vi "CleanUp.vi"(8 "error in (no error)":errorcluster, 11 "Prueba21 in":refnum<class "Prueba21.lvclass">) -> (0 "error out":errorcluster, 3 "Prueba21 out":refnum<class "Prueba21.lvclass">)   [LabVIEW 2019, in "Prueba21.lvclass"]
uses:
  Prueba21.lvclass
  C:/Users/ivan_/Documents/procal/Pruebas/Prueba/Prueba.lvclass
  Prueba/Prueba.lvclass/Prueba.ctl
  Prueba21.lvclass/Prueba21.ctl
  Base de Datos/SQLiteConnector/SQLiteConnection.lvclass
  Base de Datos/Base de Datos.lvclass
  Prueba/Prueba.lvclass
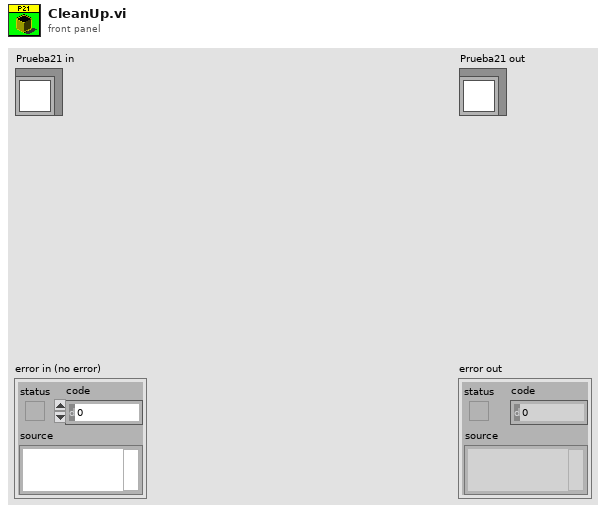
[diagram p1: front panel]
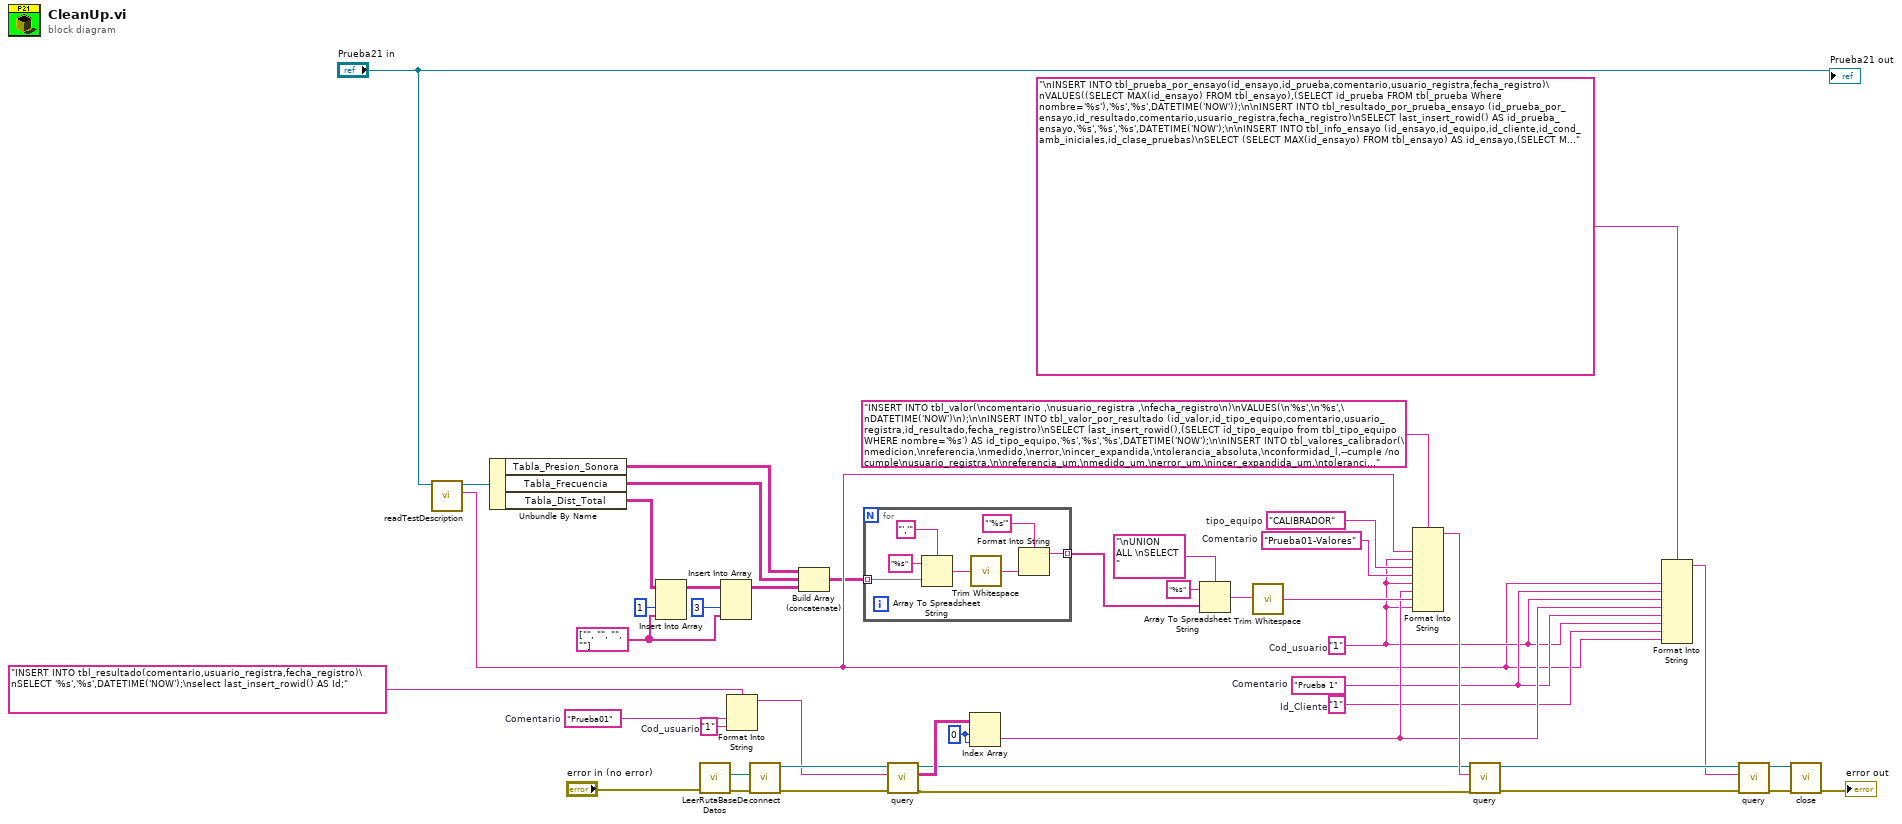
[diagram p0: block diagram]
diagram:
  w3 = string[] ["", "", "", ""]
  w18 = "1"  # Id_Cliente
  w19 = "Prueba 1"  # Comentario
  w28 = "CALIBRADOR"  # tipo_equipo
  w27 = "Prueba01-Valores"  # Comentario
  w33 = 0 ("index (row)")
  w35 = "1"  # Cod_usuario
  w36 = "Prueba01"  # Comentario
  w17 = "1"  # Cod_usuario
  n1 = call "readTestDescription.vi"("Prueba in"="Prueba21 in") -> ("Test Description"=w14:string, "Prueba out"=w15:refnum<class "Prueba21.lvclass">)  [unwired: 8 in, 1 out]
  n2 = Unbundle By Name(w15) -> ("Tabla_Presion_Sonora"=w8:string[][], "Tabla_Frecuencia"=w9:string[][], "Tabla_Dist_Total"=w2:string[][])
  n3 = Insert Into Array(array=w2, index (col)=1 ("disabled index (col)"), new element=w3) -> (w4:string[][])  [unwired: 1 in]
  n4 = call "LeerRutaBaseDeDatos.vi"("error in (no error)"="error in (no error)") -> ("error out"=w40:errorcluster, "Database Path"=w39:path)  [unwired: 9 in]
  n5 = Insert Into Array(array=w4, index (col)=3 ("disabled index (col)"), new element=w3) -> (w1:string[][])  [unwired: 1 in]
  n6 = Format Into String(format string="INSERT INTO tbl_resultado(comentario,usuario_registra,fecha_registro)\nSELECT '%s','%s',DATETIME('NOW');\nselect last_insert_rowid() AS Id;" ("SQL Statement"), w36, w35) -> (resulting string=w34:string)  [unwired: 2 in, 1 out]
  n7 = call "connect.vi"("error in (no error)"=w40, "Database Path"=w39) -> ("error out"=w32:errorcluster, "object out"=w37:refnum<class "SQLiteConnection.lvclass">)  [unwired: 8 in]
  n8 = Build Array (concatenate)(w8, w9, w1) -> (w7:string[][])
  n9 = for {
    tunnel: w7 -> [w46] mode=indexing
    tunnel: [w49] -> w43 mode=indexing
    n10 = Array To Spreadsheet String(delimiter (Tab)="','", array=w46, 3:"%s" ("format string")) -> (spreadsheet string=w48:string)
    n11 = call <vilib>:"Trim Whitespace.vi"("string"=w48) -> ("trimmed string"=w47:string)  [unwired: 1 in]
    n12 = Format Into String(format string="'%s'", w47) -> (resulting string=w49:string)  [unwired: 2 in, 1 out]
  }
  n13 = call "query.vi"("error in (no error)"=w32, "SQL Statement"=w34, "object in"=w37) -> ("error out"=w16:errorcluster, "result"=w31:string[][], "object out"=w30:refnum<class "SQLiteConnection.lvclass">)  [unwired: 5 in, 1 out]
  n14 = Index Array(array=w31, index (row)=w33, index (col)=w33) -> (element=w20:string)
  n15 = Array To Spreadsheet String(delimiter (Tab)="\nUNION ALL \nSELECT ", array=w43, 3:"%s" ("format string")) -> (spreadsheet string=w42:string)
  n16 = call <vilib>:"Trim Whitespace.vi"("string"=w42) -> ("trimmed string"=w29:string)  [unwired: 1 in]
  n17 = Format Into String(format string="INSERT INTO tbl_valor(\ncomentario ,\nusuario_registra ,\nfecha_registro\n)\nVALUES(\n'%s',\n'%s',\nDATETIME('NOW')\n);\n\nINSERT INTO tbl_valor_por_resultado (id_valor,id_tipo_equipo,comentario,usuario_registra,id_resultado,fecha_registro)\nSELECT last_insert_rowid(),(SELECT id_tipo_equipo from tbl_tipo_equipo WHERE nombre='%s') AS id_tipo_equipo,'%s','%s','%s',DATETIME('NOW');\n\nINSERT INTO tbl_valores_calibrador(\nmedicion,\nreferencia,\nmedido,\nerror,\nincer_expandida,\ntolerancia_absoluta,\nconformidad_l,--cumple /no cumple\nusuario_registra,\n\nreferencia_um,\nmedido_um,\nerror_um,\nincer_expandida_um,\ntolerancia_absoluta_um,\n\nid_valor,\nfecha_registro\n)\nSELECT * FROM(\nSELECT %s\n) AS T\nINNER JOIN\n(SELECT %s AS usuario,'dB','dB','dB','dB','dB',(SELECT MAX(id_valor) FROM tbl_valor) AS id_valor,DATETIME('NOW') fecha ) AS F;\n", w14, w17, w28, w27, w17, w20, w29, w17) -> (resulting string=w38:string)  [unwired: 2 in, 1 out]
  n18 = call "query.vi"("error in (no error)"=w16, "SQL Statement"=w38, "object in"=w30) -> ("error out"=w24:errorcluster, "object out"=w26:refnum<class "SQLiteConnection.lvclass">)  [unwired: 5 in, 2 out]
  n19 = Format Into String(format string="\nINSERT INTO tbl_prueba_por_ensayo(id_ensayo,id_prueba,comentario,usuario_registra,fecha_registro)\nVALUES((SELECT MAX(id_ensayo) FROM tbl_ensayo),(SELECT id_prueba FROM tbl_prueba Where nombre='%s'),'%s','%s',DATETIME('NOW'));\n\nINSERT INTO tbl_resultado_por_prueba_ensayo (id_prueba_por_ensayo,id_resultado,comentario,usuario_registra,fecha_registro)\nSELECT last_insert_rowid() AS id_prueba_ensayo,'%s','%s','%s',DATETIME('NOW');\n\nINSERT INTO tbl_info_ensayo (id_ensayo,id_equipo,id_cliente,id_cond_amb_iniciales,id_clase_pruebas)\nSELECT (SELECT MAX(id_ensayo) FROM tbl_ensayo) AS id_ensayo,(SELECT MAX(id_equipo) FROM tbl_equipo) AS id_equipo,'%s' AS id_cliente,(SELECT MAX(id_cond_amb_iniciales) FROM tbl_cond_amb_iniciales) AS id_cond_amb_iniciales,\n(SELECT id_clase_prueba FROM tbl_clase_prueba WHERE id_clase=(SELECT id_clase FROM tbl_equipo ORDER BY id_equipo DESC LIMIT 1)  AND id_prueba=(SELECT id_prueba FROM tbl_prueba Where nombre='%s')) AS id_clase_pruebas;\n", w14, w19, w17, w20, w19, w17, w18, w14) -> (resulting string=w21:string)  [unwired: 2 in, 1 out]
  n20 = call "query.vi"("error in (no error)"=w24, "SQL Statement"=w21, "object in"=w26) -> ("error out"=w23:errorcluster, "object out"=w25:refnum<class "SQLiteConnection.lvclass">)  [unwired: 5 in, 2 out]
  n21 = call-dynamic "close.vi"("error in (no error)"=w23, "object in"=w25) -> ("error out"=→"error out":errorcluster)  [unwired: 8 in, 1 out]
  "Prueba21 out" <- "Prueba21 in"
